vi "SLAM_constants.vi"() -> (0 "cb":dbl=0.08726646259971647, 1 "cr":dbl=0.1, 2 "landmarkDistance":dbl=0.5, 3 "maxNumberLandmarks":i32=50, 5 "CC":T1)   [LabVIEW 2009, in "LV_SLAM.lvlib"]
uses:
  LV_SLAM.lvlib
  <vilib>/Analysis/Matrix/Datatypes/RealMatrix.ctl
  <vilib>/Analysis/Matrix/Numeric/Conversions/Array To Matrix - RA2.vi
  <vilib>/Analysis/Matrix/NI_Matrix.lvlib
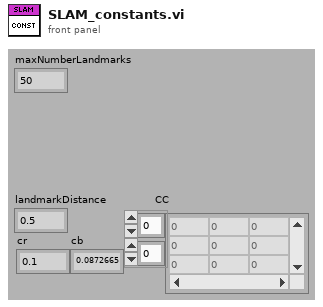
[diagram p1: front panel]
types:
  T1 = typedef "NI_Matrix.lvlib/RealMatrix.ctl" = dbl[][]
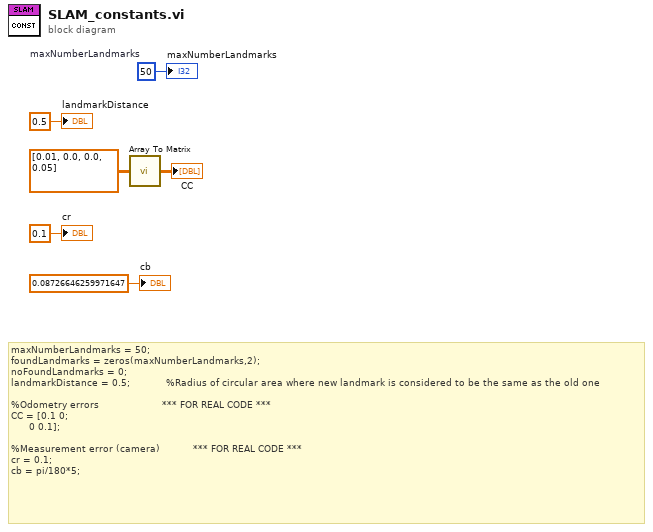
[diagram p0: block diagram]
diagram:
  w6 = 50  # maxNumberLandmarks
  # "maxNumberLandmarks = 50;\nfoundLandmarks = zeros(maxNumberLandmarks,2);\nnoFoundLandmarks = 0;\nlandmarkDistance = 0.5;            %Radius of circular area where new landmark is considered to be the same as the old one\n\n%Odometry errors                     *** FOR REAL CODE ***\nCC = [0.1 0;\n      0 0.1];\n\n%Measurement error (camera)           *** FOR REAL CODE ***\ncr = 0.1;\ncb = pi/180*5;"
  n1 = call-poly <vilib>:"Array To Matrix.vi"("Real 2D Array"=dbl[][] [[0.01, 0.0], [0.0, 0.05]] ("CC")) -> ("Real Matrix"=→"CC":T1)
  "maxNumberLandmarks" <- w6
  "landmarkDistance" <- 0.5 ("landmarkDistance")
  "cr" <- 0.1 ("cr")
  "cb" <- 0.08726646259971647 ("cb")
